vi "Send Start Command to RT Hardware's.vi"(7 "Data Cluster In":T1, 8 "error in (no error)":errorcluster) -> (0 "error out":errorcluster, 5 "Data Cluster Out":T1)   [LabVIEW 2021, in "Test Panel.lvlib"]
doc: "<b>Note:</b> This VI was modified by the <b>Validate DQMH Module</b> tool to turn off automatic error handling."
uses:
  Test Panel.lvlib
  Module Data--cluster.ctl
  GUI Ctrl Data's--Cluster.ctl
  Rx-Mapping Data.ctl
  Host-Control's/Module ID Action Enum.ctl
  Host-Control's/HW Name Enum.ctl
  <vilib>/addons/_JKI.lib/Serialization/JSON/Library/Flatten To JSON String.vi
  RT Acquisition Engine/RT Acquisition Engine.lvlib
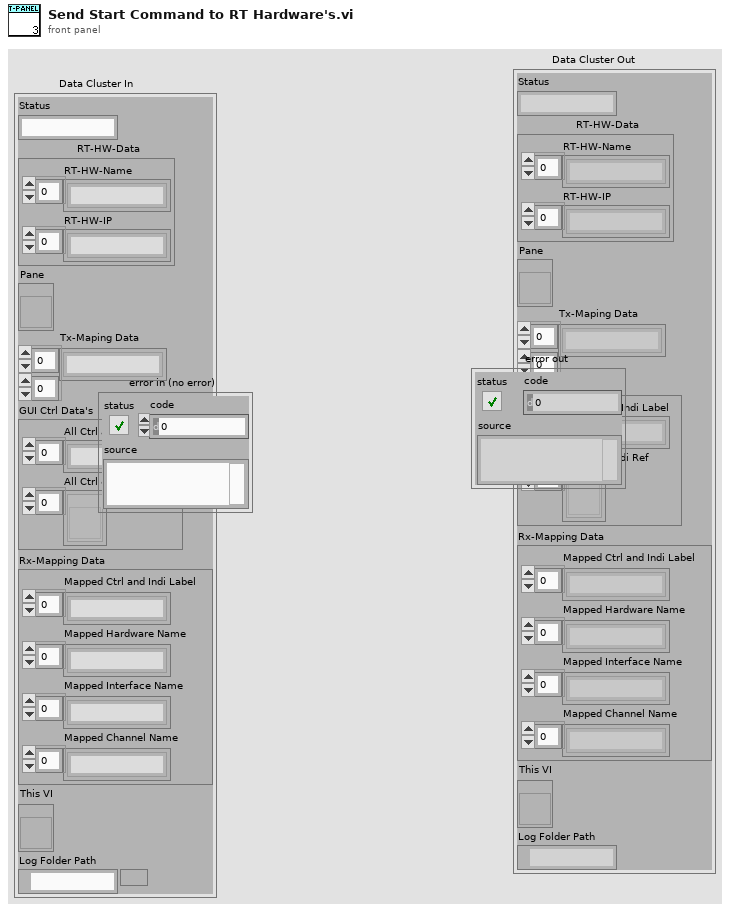
[diagram p1: front panel]
types:
  T1 = typedef "Test Panel.lvlib/Module Data--cluster.ctl" = cluster{"Status":string, "RT-HW-Data":cluster{"RT-HW-Name":string[], "RT-HW-IP":string[]}, "Pane":refnum<vi>, "Tx-Maping Data":string[][], "GUI Ctrl Data's":T2, "Rx-Mapping Data":T3, "This VI":refnum<vi>, "Log Folder Path":path}
  T2 = typedef "Test Panel.lvlib/GUI Ctrl Data's--Cluster.ctl" = cluster{"All Ctrl and Indi Label":string[], "All Ctrl & Indi Ref":refnum<vi>[]}
  T3 = typedef "Test Panel.lvlib/Rx-Mapping Data.ctl" = cluster{"Mapped Ctrl and Indi Label":string[], "Mapped Hardware Name":string[], "Mapped Interface Name":string[], "Mapped Channel Name":string[]}
  T4 = typedef "Module ID Action Enum.ctl" = enum16{"Init", "Insert", "Get a ID", "Get all ID"}
  T5 = typedef "HW Name Enum.ctl" = enum16{"Capsule-1", "Capsule-2", "Capsule-3", "Capsule-4", "sb-RIO", "Safety", "Release"}
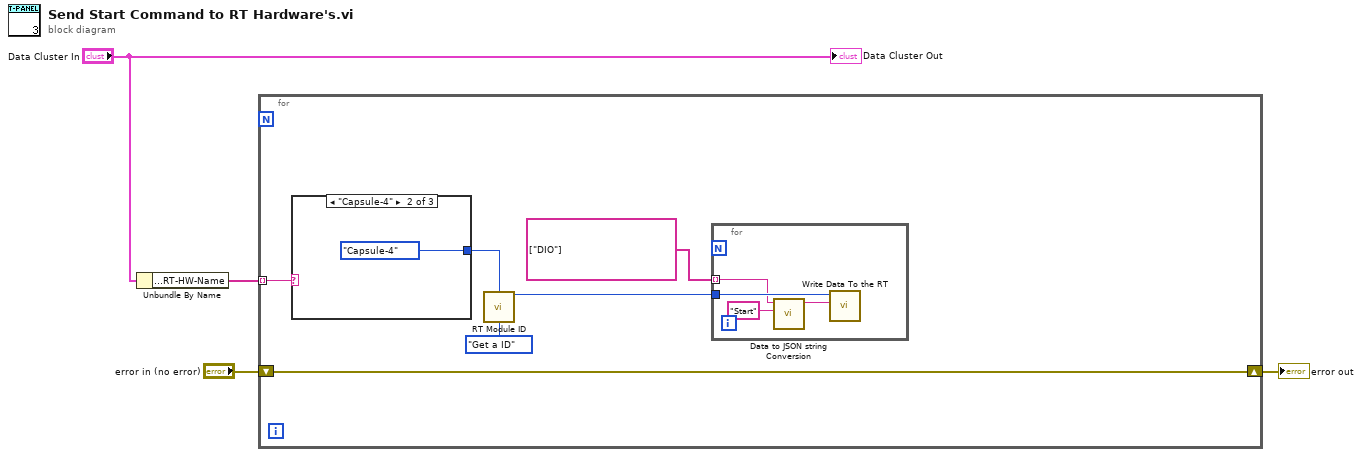
[diagram p0: block diagram]
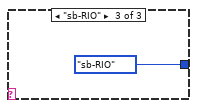
[diagram p3: hidden frame]
diagram:
  n1 = Unbundle By Name("Data Cluster In") -> ("RT-HW-Data.RT-HW-Name"=w4:string[])
  n2 = for {
    tunnel: w4 -> [w6] mode=indexing
    shift-right: [w7] -> w2
    shift-left: "error in (no error)" -> [w7]
    n3 = case shown="\"Capsule-4\"" w6 {
      tunnel: [_ HW_Name_Enum."Capsule-4" ("HW Name") HW_Name_Enum."sb-RIO" ("HW Name")] -> w8
      frame "False", Default {
      }
      frame "Capsule-4" {
      }
      frame "sb-RIO" {
      }
    }
    n4 = call "RT Module ID.vi"("HW Name"=w8, "Action"=Module_ID_Action_Enum."Get a ID") -> ("Module Id Out"=w10:i32)  [unwired: 10 in, 3 out]
    n5 = for {
      tunnel: w10 -> [w14]
      tunnel: string[] ["DIO"] ("Interface") -> [w12] mode=indexing
      n6 = call "Data to JSON string Conversion.vi"("Command"="Start", "Interface"=w12) -> ("Cmd String"=w13:string)  [unwired: 8 in, 1 out]
      n7 = call "Write Data To the RT.vi"("Data In"=w13, "Module ID"=w14) -> ()  [unwired: 9 in, 1 out]
    }
  }
  "error out" <- w2
  "Data Cluster Out" <- "Data Cluster In"
